vi "Actor Core.vi"(8 "error in":errorcluster, 11 "State in":refnum<class "Driver.lvclass">) -> (0 "error out":errorcluster, 3 "Actor out":refnum<class "Actor.lvclass">)   [LabVIEW 2013, in "Logical Systems.lvlib" / "Driver.lvlib" / "Driver.lvclass"]
doc: "(<B>Filename</B>: Actor Framework.lvlib:Actor.lvclass:Actor Core.vi)\n\nThis override invokes Entry.vi on the initial state, prior to calling the parent Actor Core. Adding this behavior to Actor Core (instead of an override of Pre Launch Init.vi) allows the initial state to launch a nested actor as part of its entry behavior.\n\nReceives messages to the actor, reacts to them, and initiates any error handling that may shut the actor down.\n\nDescendant classes may override this VI to append parallel tasks for the actor to complete while it handles messages. Overrides use the Call Parent Method node."
uses:
  Driver.lvclass
  <vilib>/ActorFramework/Actor/Actor.lvclass
  XBox Controller/Xbox Controller.ctl
  Virtual Systems/XBox Controller/XBox Controller Class/Joystick.ctl
  Driver.lvclass/Driver.ctl
  Robot Actors/System Actor/System Actor Class/System Actor.lvclass
  XBox Controller/XBox Controller Class/Xbox Controller.lvlib
panel:
  in  "Driver Status":cluster{"Current Xbox Controller":T1} {"Current Xbox Controller"."Right Joystick"."Right" min=-1.0 max=1.0 step=0.1 scale=-1.0..1.0; "Current Xbox Controller"."Right Joystick"."Forward" min=-1.0 max=1.0 step=0.1 scale=-1.0..1.0; "Current Xbox Controller"."Left Joystick"."Right" min=-1.0 max=1.0 step=0.1 scale=-1.0..1.0; "Current Xbox Controller"."Left Joystick"."Forward" min=-1.0 max=1.0 step=0.1 scale=-1.0..1.0}
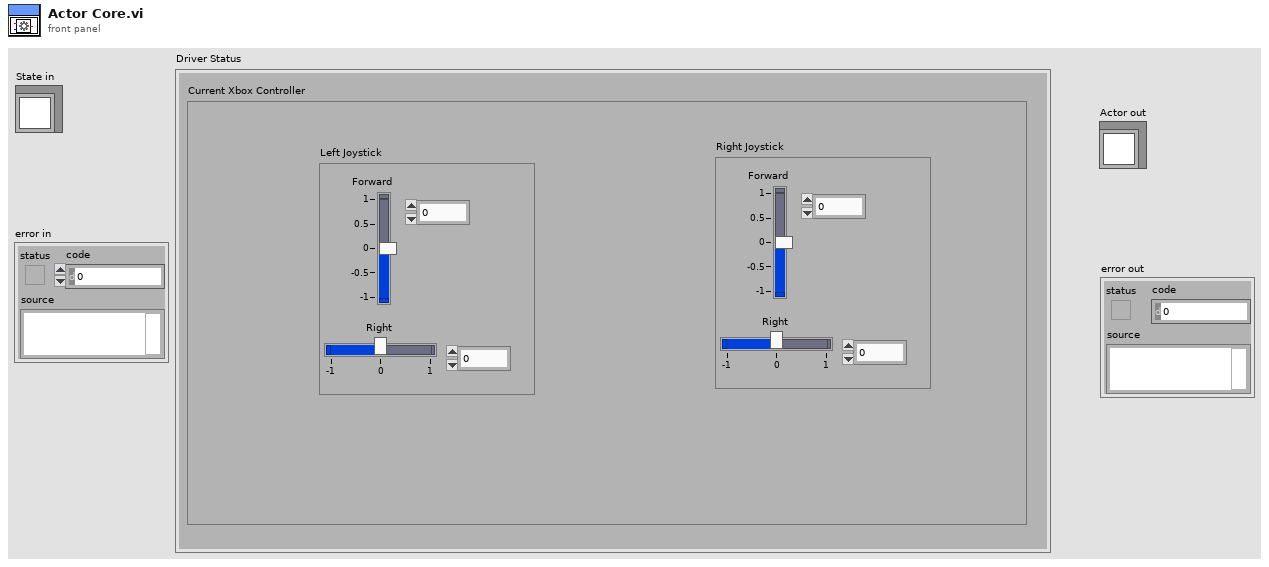
[diagram p1: front panel]
types:
  T1 = typedef "Logical Systems.lvlib/Xbox Controller.lvlib/Xbox Controller.ctl" = cluster{"Left Joystick":T2, "Right Joystick":T2}
  T2 = typedef "Logical Systems.lvlib/Xbox Controller.lvlib/Joystick.ctl" = cluster{"Forward":dbl, "Right":dbl}
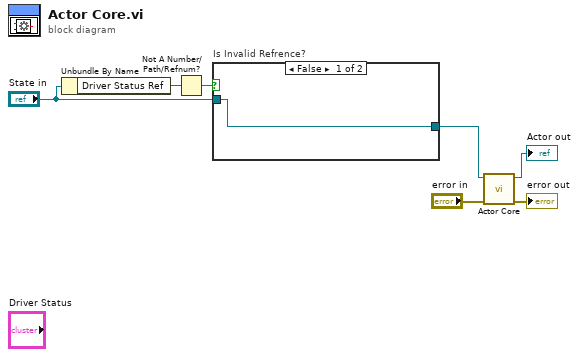
[diagram p0: block diagram]
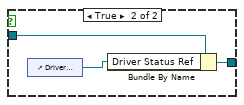
[diagram p2: hidden frame]
diagram:
  n1 = Unbundle By Name("State in") -> ("Driver Status Ref"=w4:refnum<vi>)
  n2 = Not A Number/Path/Refnum?(number/path/refnum=w4) -> (NaN/Path/Refnum?=w3:bool)
  n3 = case "Is Invalid Refrence?" shown="False" w3 {
    tunnel: "State in" -> [w8 w11]
    tunnel: [w8 w10] -> w1
    frame False {
    }
    frame True {
      n4 = control-ref of="Driver Status"() -> (w9:refnum<vi>)
      n5 = Bundle By Name(cluster=w11, "Driver Status Ref"=w9) -> (w10:refnum<class "Driver.lvclass">)
    }
  }
  n6 = call-parent "Actor Core.vi"("error in"="error in", "State in"=w1) -> ("error out"=→"error out":errorcluster, "Actor out"=→"Actor out":refnum<class "Actor.lvclass">)  [unwired: 8 in]
